vi "Robot_Control.vi"() -> ()   [LabVIEW 2014]
uses:
  <vilib>/LabVIEW Targets/FPGA/cRIO/cRIO-9505/controls.llb/_nicrio_cRIO-9505_DriveDirection.ctl
  <vilib>/Platform/TimedLoop/XDataNode/timing_clust.ctl
  <vilib>/Platform/TimedLoop/XDataNode/nitl_modes.ctl
  <vilib>/Platform/TimedLoop/XDataNode/wakeup.ctl
  <vilib>/rvi/Emulation/niFpgaGetClockAttributes.vi
  <vilib>/rvi/Emulation/niFpgaSctlEmulationGetInTimedLoop.vi
  <vilib>/rvi/Emulation/niFpgaEmulationReportErrorSimple.vi
  <vilib>/rvi/eio/common/nirviEmuTemplateMethod_errors.vi
  <vilib>/rvi/Emulation/niFpgaCriticalErrorInLSC.vi
  <vilib>/rvi/Emulation/niFpgaProcessEmulError.vi
  <vilib>/eio/EIONode/EIONode.xnode
  <vilib>/eio/EIOMethodNode/EIOMethodNode.xnode
  <vilib>/Platform/TimedLoop/XDataNode/XDataNode.xnode
  <vilib>/Platform/TimedLoop/XDataNode/XDNodeRunTimeDep.lvlib
panel:
  out "Mod1 6/Current Sense":i16
  in  "Duty Cycle 6":fxp<+,32,0>=0.5
  in  "Mod1/Drive Direction 6":T1
  out "Boolean 5":bool
  out "Boolean 4":bool
  out "Boolean 3":bool
  out "Boolean 2":bool
  out "Boolean":bool
  in  "Velocity Interval (uSec)":fxp<+/-,40,24>=5000.0
  out "Homed":bool
  in  "Duty Cycle 5":fxp<+,32,0>=0.5
  in  "Duty Cycle 4":fxp<+,32,0>=0.5
  in  "Duty Cycle 3":fxp<+,32,0>=0.5
  in  "Duty Cycle 2":fxp<+,32,0>=0.5
  in  "Duty Cycle 1":fxp<+,32,0>=0.5
  in  "Stop":bool
  in  "Mod1/Drive Direction 5":T1
  in  "Mod1/Drive Direction 4":T1=enum."Counterclockwise"
  in  "Mod1/Drive Direction 3":T1=enum."Counterclockwise"
  in  "Mod1/Drive Direction 2":T1=enum."Counterclockwise"
  in  "Mod1/Drive Direction":T1
  out "Position (Degrees) 5":fxp<+/-,40,24>
  out "Velocity (Degrees/Second) 5":fxp<+/-,40,24>
  out "Position (Degrees) 4":fxp<+/-,40,24>
  out "Velocity (Degrees/Second) 4":fxp<+/-,40,24>
  out "Position (Degrees) 3":fxp<+/-,40,24>
  out "Velocity (Degrees/Second) 3":fxp<+/-,40,24>
  out "Position (Degrees) 2":fxp<+/-,40,24>
  out "Velocity (Degrees/Second) 2":fxp<+/-,40,24>
  in  "Go":bool
  out "Velocity (Degrees/Second)":fxp<+/-,40,24>
  out "Position (Degrees)":fxp<+/-,40,24>
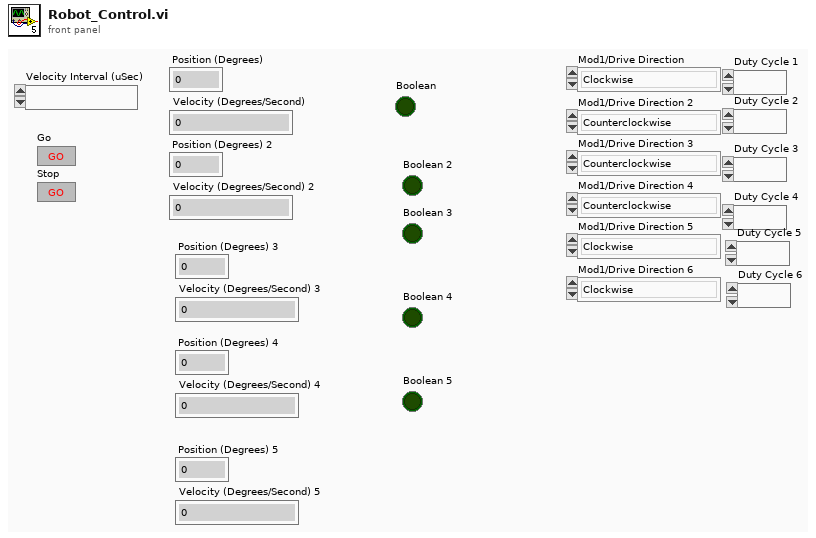
[diagram p1: front panel]
types:
  T1 = typedef "_nicrio_cRIO-9505_DriveDirection.ctl" = enum8{"Clockwise", "Counterclockwise"}
  T2 = typedef "XDNodeRunTimeDep.lvlib/timing_clust.ctl" = cluster{"Expected End [f-1]":u64, "Actual End [f-1]":u64, "Finished Late? [f-1]":bool, "Expected End [i-1]":u64, "Actual End [i-1]":u64, "Finished Late? [i-1]":bool, "Expected Start [i]":u64, "Actual Start [i]":u64, "Expected Start [f]":u64, "Actual Start [f]":u64, "Source Name":string, "Structure Name":string, "Period":i64, "Deadline":i64, "Offset":i64, "Start":i64, "Priority":i32, "Timeout":i32, "Mode":T3, "Wakeup Reason":T4, "Error":errorcluster, "Source Type":string, "Secondary Source Type":string, "Global End Time":u64, "Global Start Time":u64, "Frame Duration":u64, "Iteration Duration":u64, "Assigned CPU":i32, "I/O Scan Engine Mode":u32}
  T3 = typedef "XDNodeRunTimeDep.lvlib/nitl_modes.ctl" = enum32{"No Change", "Process missed periods, maintain original phase", "Discard missed periods, maintain original phase", "Process missed periods, ignore original phase", "Discard missed periods, ignore original phase"}
  T4 = typedef "XDNodeRunTimeDep.lvlib/wakeup.ctl" = enum32{"Normal", "Aborted", "Asynchronous wakeup", "Timing source error", "Timed loop error", "Timeout"}
  T5 = cluster{"A'":bool, "B'":bool, "Time Interval Reached":bool, "Reference Time Count":fxp<+/-,40,24>, "Previous Tick Count":fxp<+/-,40,24>, "Previous Interval Tick Count":fxp<+/-,40,24>, "Velocity":fxp<+/-,40,24>}
  T6 = cluster{"A'":bool, "B'":bool, "Time Interval Reached":bool, "Reference Time Count":fxp<+/-,64,64>, "Previous Tick Count":fxp<+/-,40,24>, "Previous Interval Tick Count":fxp<+/-,40,24>, "Velocity":fxp<+/-,40,24>}
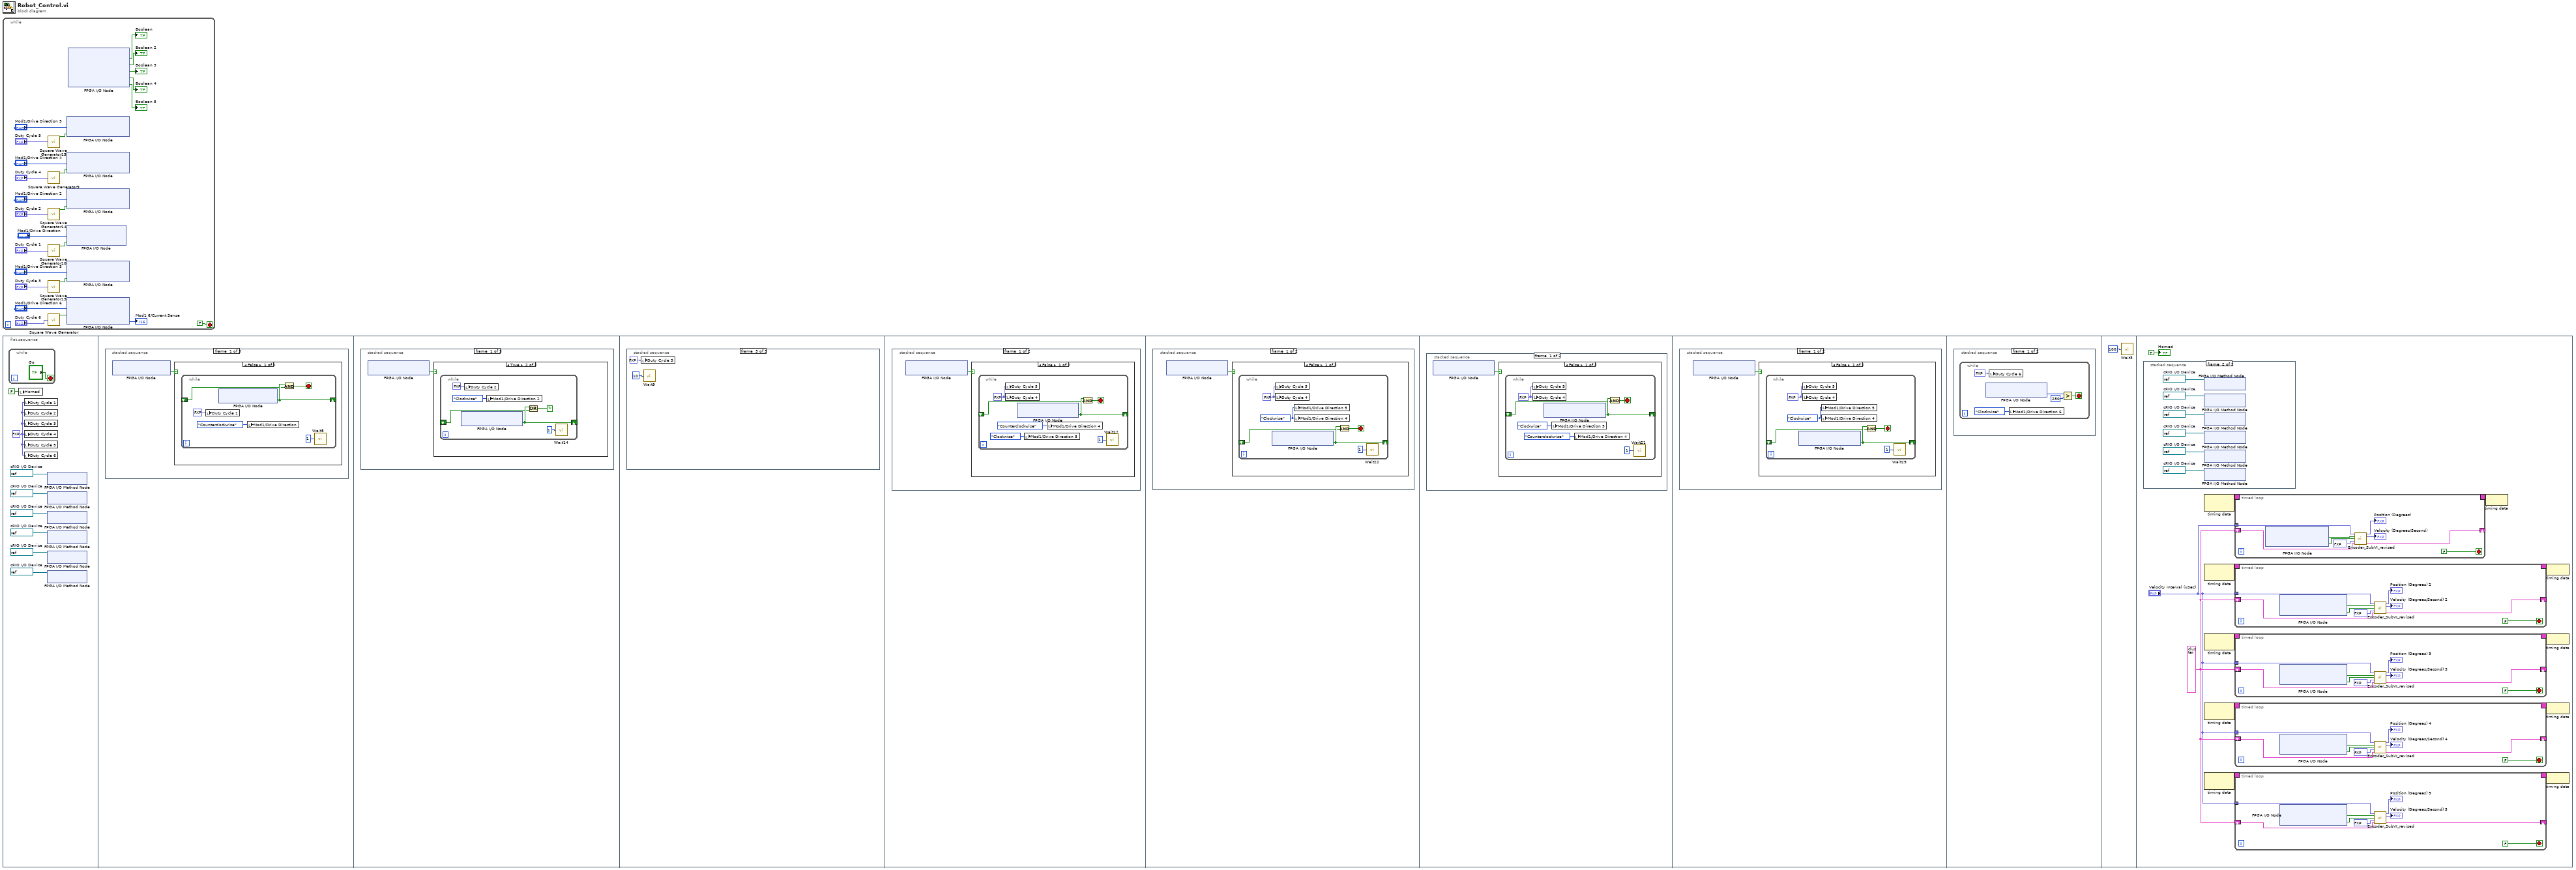
[diagram p0: block diagram]
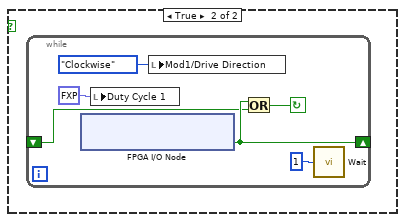
[diagram p2: hidden frame]
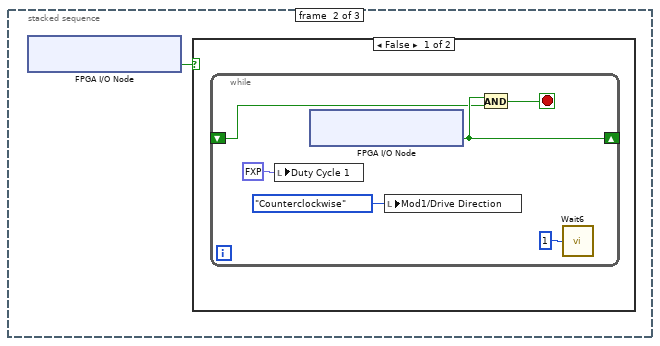
[diagram p3: hidden frame]
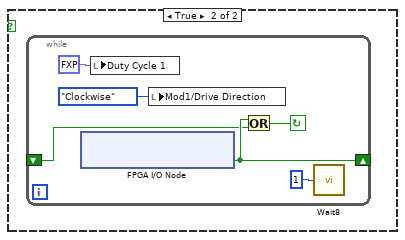
[diagram p4: hidden frame]
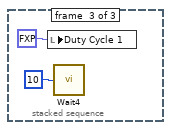
[diagram p5: hidden frame]
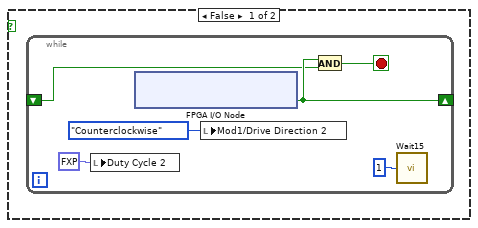
[diagram p6: hidden frame]
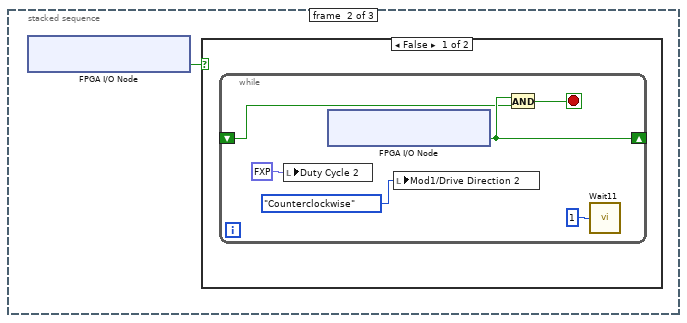
[diagram p7: hidden frame]
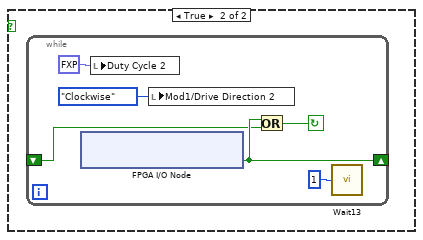
[diagram p8: hidden frame]
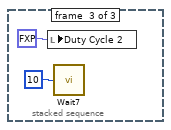
[diagram p9: hidden frame]
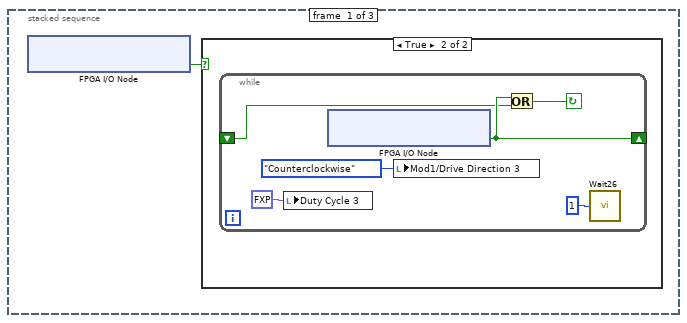
[diagram p10: hidden frame]
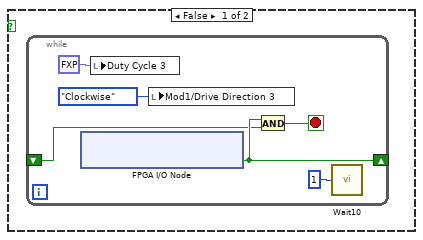
[diagram p11: hidden frame]
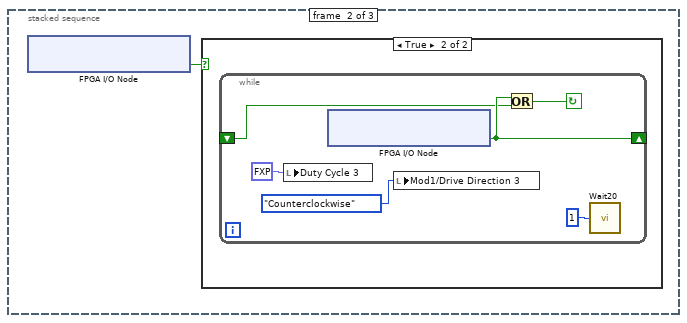
[diagram p12: hidden frame]
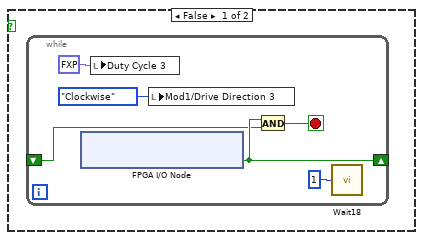
[diagram p13: hidden frame]
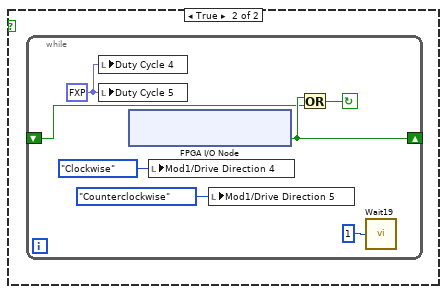
[diagram p14: hidden frame]
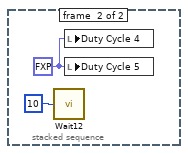
[diagram p15: hidden frame]
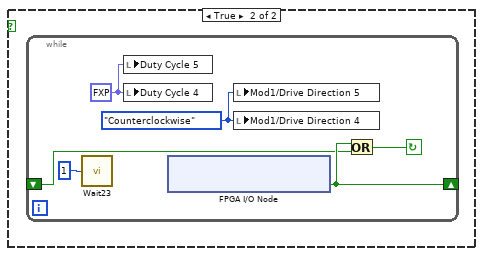
[diagram p16: hidden frame]
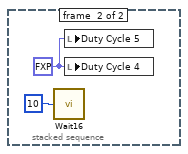
[diagram p17: hidden frame]
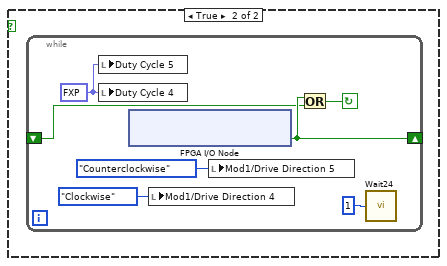
[diagram p18: hidden frame]
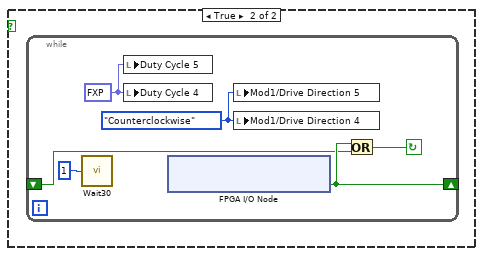
[diagram p20: hidden frame]
diagram:
  n1 = while {
    stop <- FALSE stop-if-true
    n2 = call "Square Wave Generator15"("duty cycle (periods)"="Duty Cycle 5") -> ("square wave out"=w2:bool)  [unwired: 14 in]
    n3 = call "Square Wave Generator9"("duty cycle (periods)"="Duty Cycle 4") -> ("square wave out"=w17:bool)  [unwired: 14 in]
    n4 = call "Square Wave Generator14"("duty cycle (periods)"="Duty Cycle 2") -> ("square wave out"=w3:bool)  [unwired: 14 in]
    n5 = call "Square Wave Generator10"("duty cycle (periods)"="Duty Cycle 1") -> ("square wave out"=w16:bool)  [unwired: 14 in]
    n6 = call "Square Wave Generator13"("duty cycle (periods)"="Duty Cycle 3") -> ("square wave out"=w4:bool)  [unwired: 14 in]
    n7 = call "Square Wave Generator"("duty cycle (periods)"="Duty Cycle 6") -> ("square wave out"=w18:bool)  [unwired: 14 in]
    n8 = xnode "FPGA I/O Node"("Mod1 5/Drive Direction"="Mod1/Drive Direction 5", "Mod1 5/Motor"=w2) -> ()  [unwired: 2 in, 2 out]
    n9 = xnode "FPGA I/O Node"("Mod1 4/Drive Direction"="Mod1/Drive Direction 4", "Mod1 4/Motor"=w17) -> ()  [unwired: 2 in, 2 out]
    n10 = xnode "FPGA I/O Node"("Mod1 2/Drive Direction"="Mod1/Drive Direction 2", "Mod1 2/Motor"=w3) -> ()  [unwired: 2 in, 2 out]
    n11 = xnode "FPGA I/O Node"("Mod1/Drive Direction"="Mod1/Drive Direction", "Mod1/Motor"=w16) -> ()  [unwired: 2 in, 2 out]
    n12 = xnode "FPGA I/O Node"("Mod1 3/Drive Direction"="Mod1/Drive Direction 3", "Mod1 3/Motor"=w4) -> ()  [unwired: 2 in, 2 out]
    n13 = xnode "FPGA I/O Node"("Mod1 6/Drive Direction"="Mod1/Drive Direction 6", "Mod1 6/Motor"=w18) -> ("Mod1 6/Current Sense"=→"Mod1 6/Current Sense":i16)  [unwired: 3 in, 3 out]
    n14 = xnode "FPGA I/O Node"() -> ("Mod1/Encoder Index"=→"Boolean":bool, "Mod1 2/Encoder Index"=→"Boolean 2":bool, "Mod1 3/Encoder Index"=→"Boolean 3":bool, "Mod1 4/Encoder Index"=→"Boolean 4":bool, "Mod1 5/Encoder Index"=→"Boolean 5":bool)  [unwired: 5 in, 5 out]
  }
  n15 = flat-sequence {
    frame #0 {
      w27 = refnum<k21> "Mod6"  # cRIO I/O Device
      w26 = fxp<+,32,0> 0.0 ("Duty Cycle 1")
      w31 = refnum<k21> "Mod5"  # cRIO I/O Device
      w30 = refnum<k21> "Mod4"  # cRIO I/O Device
      w29 = refnum<k21> "Mod3"  # cRIO I/O Device
      w32 = refnum<k21> "Mod2"  # cRIO I/O Device
      w33 = refnum<k21> "Mod1"  # cRIO I/O Device
      n16 = while {
        stop <- "Go" stop-if-true
      }
      n17 = local write "Homed"(FALSE ("Homed")) -> ()
      n18 = local write "Duty Cycle 1"(w26) -> ()
      n19 = local write "Duty Cycle 2"(w26) -> ()
      n20 = local write "Duty Cycle 3"(w26) -> ()
      n21 = local write "Duty Cycle 4"(w26) -> ()
      n22 = local write "Duty Cycle 5"(w26) -> ()
      n23 = local write "Duty Cycle 6"(w26) -> ()
      n24 = xnode "FPGA I/O Method Node"("FPGA I/O In"=w33) -> ()  [unwired: 1 out]
      n25 = xnode "FPGA I/O Method Node"("FPGA I/O In"=w32) -> ()  [unwired: 1 out]
      n26 = xnode "FPGA I/O Method Node"("FPGA I/O In"=w29) -> ()  [unwired: 1 out]
      n27 = xnode "FPGA I/O Method Node"("FPGA I/O In"=w30) -> ()  [unwired: 1 out]
      n28 = xnode "FPGA I/O Method Node"("FPGA I/O In"=w27) -> ()  [unwired: 1 out]
      n29 = xnode "FPGA I/O Method Node"("FPGA I/O In"=w31) -> ()  [unwired: 1 out]
    }
    frame #1 {
      n30 = stacked-sequence {
        frame #0 {
          n31 = xnode "FPGA I/O Node"() -> ("Mod1/Encoder Index"=w35:bool)  [unwired: 1 in, 1 out]
          n32 = case shown="False" w35 {
            frame False {
              n33 = while {
                shift-right: [w37] -> _
                shift-left: _ -> [w36]
                stop <- w38 stop-if-true
                n34 = local write "Duty Cycle 1"(fxp<+,32,0> 0.6999999999534339 ("phase offset (periods)")) -> ()
                n35 = xnode "FPGA I/O Node"() -> ("Mod1/Encoder Index"=w37:bool)  [unwired: 1 in, 1 out]
                n36 = local write "Mod1/Drive Direction"(_nicrio_cRIO-9505_DriveDirection."Counterclockwise" ("Mod1/Drive Direction")) -> ()
                n37 = And(x=w37, y=w36) -> (x .and. y?=w38:bool)
                n38 = call "Wait5"("Count(mSec)"=u32 1) -> ()  [unwired: 1 out]
              }
            }
            frame True {
              n39 = while {
                shift-right: [w43] -> _
                shift-left: _ -> [w42]
                stop <- w44 continue-if-true
                n40 = xnode "FPGA I/O Node"() -> ("Mod1/Encoder Index"=w43:bool)  [unwired: 1 in, 1 out]
                n41 = local write "Duty Cycle 1"(fxp<+,32,0> 0.6999999999534339 ("phase offset (periods)")) -> ()
                n42 = local write "Mod1/Drive Direction"(_nicrio_cRIO-9505_DriveDirection."Clockwise" ("Mod1/Drive Direction")) -> ()
                n43 = Or(x=w43, y=w42) -> (x .or. y?=w44:bool)
                n44 = call "Wait"("Count(mSec)"=u32 1) -> ()  [unwired: 1 out]
              }
            }
          }
        }
        frame #1 {
          n45 = xnode "FPGA I/O Node"() -> ("Mod1/Encoder Index"=w48:bool)  [unwired: 1 in, 1 out]
          n46 = case shown="False" w48 {
            frame False {
              n47 = while {
                shift-right: [w50] -> _
                shift-left: _ -> [w49]
                stop <- w51 stop-if-true
                n48 = local write "Duty Cycle 1"(fxp<+,32,0> 0.19999999995343387 ("phase offset (periods)")) -> ()
                n49 = xnode "FPGA I/O Node"() -> ("Mod1/Encoder Index"=w50:bool)  [unwired: 1 in, 1 out]
                n50 = local write "Mod1/Drive Direction"(_nicrio_cRIO-9505_DriveDirection."Counterclockwise" ("Mod1/Drive Direction")) -> ()
                n51 = And(x=w50, y=w49) -> (x .and. y?=w51:bool)
                n52 = call "Wait6"("Count(mSec)"=u32 1) -> ()  [unwired: 1 out]
              }
            }
            frame True {
              n53 = while {
                shift-right: [w56] -> _
                shift-left: _ -> [w55]
                stop <- w57 continue-if-true
                n54 = xnode "FPGA I/O Node"() -> ("Mod1/Encoder Index"=w56:bool)  [unwired: 1 in, 1 out]
                n55 = local write "Duty Cycle 1"(fxp<+,32,0> 0.19999999995343387 ("phase offset (periods)")) -> ()
                n56 = local write "Mod1/Drive Direction"(_nicrio_cRIO-9505_DriveDirection."Clockwise" ("Mod1/Drive Direction")) -> ()
                n57 = Or(x=w56, y=w55) -> (x .or. y?=w57:bool)
                n58 = call "Wait8"("Count(mSec)"=u32 1) -> ()  [unwired: 1 out]
              }
            }
          }
        }
        frame #2 {
          n59 = local write "Duty Cycle 1"(fxp<+,32,0> 0.0 ("Duty Cycle 1")) -> ()
          n60 = call "Wait4"("Count(mSec)"=u32 10) -> ()  [unwired: 1 out]
        }
      }
    }
    frame #2 {
      n61 = stacked-sequence {
        frame #0 {
          n62 = xnode "FPGA I/O Node"() -> ("Mod1 2/Encoder Index"=w63:bool)  [unwired: 1 in, 1 out]
          n63 = case shown="True" w63 {
            frame False {
              n64 = while {
                shift-right: [w65] -> _
                shift-left: _ -> [w64]
                stop <- w66 stop-if-true
                n65 = local write "Duty Cycle 2"(fxp<+,32,0> 0.6999999999534339 ("phase offset (periods)")) -> ()
                n66 = xnode "FPGA I/O Node"() -> ("Mod1 2/Encoder Index"=w65:bool)  [unwired: 1 in, 1 out]
                n67 = local write "Mod1/Drive Direction 2"(_nicrio_cRIO-9505_DriveDirection."Counterclockwise" ("Mod1/Drive Direction")) -> ()
                n68 = And(x=w65, y=w64) -> (x .and. y?=w66:bool)
                n69 = call "Wait15"("Count(mSec)"=u32 1) -> ()  [unwired: 1 out]
              }
            }
            frame True {
              n70 = while {
                shift-right: [w71] -> _
                shift-left: _ -> [w70]
                stop <- w72 continue-if-true
                n71 = xnode "FPGA I/O Node"() -> ("Mod1 2/Encoder Index"=w71:bool)  [unwired: 1 in, 1 out]
                n72 = local write "Duty Cycle 2"(fxp<+,32,0> 0.6999999999534339 ("phase offset (periods)")) -> ()
                n73 = local write "Mod1/Drive Direction 2"(_nicrio_cRIO-9505_DriveDirection."Clockwise" ("Mod1/Drive Direction")) -> ()
                n74 = Or(x=w71, y=w70) -> (x .or. y?=w72:bool)
                n75 = call "Wait14"("Count(mSec)"=u32 1) -> ()  [unwired: 1 out]
              }
            }
          }
        }
        frame #1 {
          n76 = xnode "FPGA I/O Node"() -> ("Mod1 2/Encoder Index"=w76:bool)  [unwired: 1 in, 1 out]
          n77 = case shown="False" w76 {
            frame False {
              n78 = while {
                shift-right: [w78] -> _
                shift-left: _ -> [w77]
                stop <- w79 stop-if-true
                n79 = local write "Duty Cycle 2"(fxp<+,32,0> 0.19999999995343387 ("phase offset (periods)")) -> ()
                n80 = xnode "FPGA I/O Node"() -> ("Mod1 2/Encoder Index"=w78:bool)  [unwired: 1 in, 1 out]
                n81 = local write "Mod1/Drive Direction 2"(_nicrio_cRIO-9505_DriveDirection."Counterclockwise" ("Mod1/Drive Direction")) -> ()
                n82 = And(x=w78, y=w77) -> (x .and. y?=w79:bool)
                n83 = call "Wait11"("Count(mSec)"=u32 1) -> ()  [unwired: 1 out]
              }
            }
            frame True {
              n84 = while {
                shift-right: [w84] -> _
                shift-left: _ -> [w83]
                stop <- w85 continue-if-true
                n85 = xnode "FPGA I/O Node"() -> ("Mod1 2/Encoder Index"=w84:bool)  [unwired: 1 in, 1 out]
                n86 = local write "Duty Cycle 2"(fxp<+,32,0> 0.19999999995343387 ("phase offset (periods)")) -> ()
                n87 = local write "Mod1/Drive Direction 2"(_nicrio_cRIO-9505_DriveDirection."Clockwise" ("Mod1/Drive Direction")) -> ()
                n88 = Or(x=w84, y=w83) -> (x .or. y?=w85:bool)
                n89 = call "Wait13"("Count(mSec)"=u32 1) -> ()  [unwired: 1 out]
              }
            }
          }
        }
        frame #2 {
          n90 = local write "Duty Cycle 2"(fxp<+,32,0> 0.0 ("Duty Cycle 2")) -> ()
          n91 = call "Wait7"("Count(mSec)"=u32 10) -> ()  [unwired: 1 out]
        }
      }
    }
    frame #3 {
      n92 = stacked-sequence {
        frame #0 {
          n93 = xnode "FPGA I/O Node"() -> ("Mod1 3/Encoder Index"=w91:bool)  [unwired: 1 in, 1 out]
          n94 = case shown="True" w91 {
            frame False {
              n95 = while {
                shift-right: [w93] -> _
                shift-left: _ -> [w92]
                stop <- w94 stop-if-true
                n96 = xnode "FPGA I/O Node"() -> ("Mod1 3/Encoder Index"=w93:bool)  [unwired: 1 in, 1 out]
                n97 = local write "Duty Cycle 3"(fxp<+,32,0> 0.6999999999534339 ("phase offset (periods)")) -> ()
                n98 = local write "Mod1/Drive Direction 3"(_nicrio_cRIO-9505_DriveDirection."Clockwise" ("Mod1/Drive Direction")) -> ()
                n99 = And(x=w93, y=w92) -> (x .and. y?=w94:bool)
                n100 = call "Wait10"("Count(mSec)"=u32 1) -> ()  [unwired: 1 out]
              }
            }
            frame True {
              n101 = while {
                shift-right: [w99] -> _
                shift-left: _ -> [w98]
                stop <- w100 continue-if-true
                n102 = local write "Duty Cycle 3"(fxp<+,32,0> 0.6999999999534339 ("phase offset (periods)")) -> ()
                n103 = xnode "FPGA I/O Node"() -> ("Mod1 3/Encoder Index"=w99:bool)  [unwired: 1 in, 1 out]
                n104 = local write "Mod1/Drive Direction 3"(_nicrio_cRIO-9505_DriveDirection."Counterclockwise" ("Mod1/Drive Direction")) -> ()
                n105 = Or(x=w99, y=w98) -> (x .or. y?=w100:bool)
                n106 = call "Wait26"("Count(mSec)"=u32 1) -> ()  [unwired: 1 out]
              }
            }
          }
        }
        frame #1 {
          n107 = xnode "FPGA I/O Node"() -> ("Mod1 3/Encoder Index"=w104:bool)  [unwired: 1 in, 1 out]
          n108 = case shown="True" w104 {
            frame False {
              n109 = while {
                shift-right: [w106] -> _
                shift-left: _ -> [w105]
                stop <- w107 stop-if-true
                n110 = xnode "FPGA I/O Node"() -> ("Mod1 3/Encoder Index"=w106:bool)  [unwired: 1 in, 1 out]
                n111 = local write "Duty Cycle 3"(fxp<+,32,0> 0.19999999995343387 ("phase offset (periods)")) -> ()
                n112 = local write "Mod1/Drive Direction 3"(_nicrio_cRIO-9505_DriveDirection."Clockwise" ("Mod1/Drive Direction")) -> ()
                n113 = And(x=w106, y=w105) -> (x .and. y?=w107:bool)
                n114 = call "Wait18"("Count(mSec)"=u32 1) -> ()  [unwired: 1 out]
              }
            }
            frame True {
              n115 = while {
                shift-right: [w112] -> _
                shift-left: _ -> [w111]
                stop <- w113 continue-if-true
                n116 = local write "Duty Cycle 3"(fxp<+,32,0> 0.19999999995343387 ("phase offset (periods)")) -> ()
                n117 = xnode "FPGA I/O Node"() -> ("Mod1 3/Encoder Index"=w112:bool)  [unwired: 1 in, 1 out]
                n118 = local write "Mod1/Drive Direction 3"(_nicrio_cRIO-9505_DriveDirection."Counterclockwise" ("Mod1/Drive Direction")) -> ()
                n119 = Or(x=w112, y=w111) -> (x .or. y?=w113:bool)
                n120 = call "Wait20"("Count(mSec)"=u32 1) -> ()  [unwired: 1 out]
              }
            }
          }
        }
        frame #2 {
          n121 = local write "Duty Cycle 3"(fxp<+,32,0> 0.0 ("Duty Cycle 3")) -> ()
          n122 = call "Wait9"("Count(mSec)"=u32 10) -> ()  [unwired: 1 out]
        }
      }
    }
    frame #4 {
      n123 = stacked-sequence {
        frame #0 {
          n124 = xnode "FPGA I/O Node"() -> ("Mod1 4/Encoder Index"=w119:bool)  [unwired: 1 in, 1 out]
          n125 = case shown="False" w119 {
            frame False {
              n126 = while {
                shift-right: [w121] -> _
                shift-left: _ -> [w120]
                stop <- w122 stop-if-true
                w125 = fxp<+,32,0> 0.6999999999534339 ("phase offset (periods)")
                n127 = local write "Duty Cycle 5"(w125) -> ()
                n128 = local write "Duty Cycle 4"(w125) -> ()
                n129 = xnode "FPGA I/O Node"() -> ("Mod1 4/Encoder Index"=w121:bool)  [unwired: 1 in, 1 out]
                n130 = local write "Mod1/Drive Direction 5"(_nicrio_cRIO-9505_DriveDirection."Clockwise" ("Mod1/Drive Direction")) -> ()
                n131 = local write "Mod1/Drive Direction 4"(_nicrio_cRIO-9505_DriveDirection."Counterclockwise" ("Mod1/Drive Direction")) -> ()
                n132 = And(x=w121, y=w120) -> (x .and. y?=w122:bool)
                n133 = call "Wait17"("Count(mSec)"=u32 1) -> ()  [unwired: 1 out]
              }
            }
            frame True {
              n134 = while {
                shift-right: [w128] -> _
                shift-left: _ -> [w127]
                stop <- w129 continue-if-true
                w130 = fxp<+,32,0> 0.6999999999534339 ("phase offset (periods)")
                n135 = local write "Duty Cycle 4"(w130) -> ()
                n136 = local write "Duty Cycle 5"(w130) -> ()
                n137 = xnode "FPGA I/O Node"() -> ("Mod1 4/Encoder Index"=w128:bool)  [unwired: 1 in, 1 out]
                n138 = local write "Mod1/Drive Direction 4"(_nicrio_cRIO-9505_DriveDirection."Clockwise" ("Mod1/Drive Direction")) -> ()
                n139 = local write "Mod1/Drive Direction 5"(_nicrio_cRIO-9505_DriveDirection."Counterclockwise" ("Mod1/Drive Direction")) -> ()
                n140 = Or(x=w128, y=w127) -> (x .or. y?=w129:bool)
                n141 = call "Wait19"("Count(mSec)"=u32 1) -> ()  [unwired: 1 out]
              }
            }
          }
        }
        frame #1 {
          w135 = fxp<+,32,0> 0.0 ("Duty Cycle 4")
          n142 = call "Wait12"("Count(mSec)"=u32 10) -> ()  [unwired: 1 out]
          n143 = local write "Duty Cycle 4"(w135) -> ()
          n144 = local write "Duty Cycle 5"(w135) -> ()
        }
      }
    }
    frame #5 {
      n145 = stacked-sequence {
        frame #0 {
          n146 = xnode "FPGA I/O Node"() -> ("Mod1 5/Encoder Index"=w136:bool)  [unwired: 1 in, 1 out]
          n147 = case shown="False" w136 {
            frame False {
              n148 = while {
                shift-right: [w139] -> _
                shift-left: _ -> [w137]
                stop <- w138 stop-if-true
                w140 = fxp<+,32,0> 0.6999999999534339 ("phase offset (periods)")
                w142 = _nicrio_cRIO-9505_DriveDirection."Clockwise" ("Mod1/Drive Direction")
                n149 = xnode "FPGA I/O Node"() -> ("Mod1 5/Encoder Index"=w139:bool)  [unwired: 1 in, 1 out]
                n150 = local write "Duty Cycle 5"(w140) -> ()
                n151 = local write "Duty Cycle 4"(w140) -> ()
                n152 = local write "Mod1/Drive Direction 5"(w142) -> ()
                n153 = local write "Mod1/Drive Direction 4"(w142) -> ()
                n154 = And(x=w139, y=w137) -> (x .and. y?=w138:bool)
                n155 = call "Wait22"("Count(mSec)"=u32 1) -> ()  [unwired: 1 out]
              }
            }
            frame True {
              n156 = while {
                shift-right: [w144] -> _
                shift-left: _ -> [w143]
                stop <- w145 continue-if-true
                w146 = fxp<+,32,0> 0.6999999999534339 ("phase offset (periods)")
                w148 = _nicrio_cRIO-9505_DriveDirection."Counterclockwise" ("Mod1/Drive Direction")
                n157 = call "Wait23"("Count(mSec)"=u32 1) -> ()  [unwired: 1 out]
                n158 = local write "Duty Cycle 5"(w146) -> ()
                n159 = local write "Duty Cycle 4"(w146) -> ()
                n160 = xnode "FPGA I/O Node"() -> ("Mod1 5/Encoder Index"=w144:bool)  [unwired: 1 in, 1 out]
                n161 = local write "Mod1/Drive Direction 5"(w148) -> ()
                n162 = local write "Mod1/Drive Direction 4"(w148) -> ()
                n163 = Or(x=w144, y=w143) -> (x .or. y?=w145:bool)
              }
            }
          }
        }
        frame #1 {
          w150 = fxp<+,32,0> 0.0 ("Duty Cycle 4")
          n164 = call "Wait16"("Count(mSec)"=u32 10) -> ()  [unwired: 1 out]
          n165 = local write "Duty Cycle 5"(w150) -> ()
          n166 = local write "Duty Cycle 4"(w150) -> ()
        }
      }
    }
    frame #6 {
      n167 = stacked-sequence {
        frame #0 {
          n168 = xnode "FPGA I/O Node"() -> ("Mod1 4/Encoder Index"=w151:bool)  [unwired: 1 in, 1 out]
          n169 = case shown="False" w151 {
            frame False {
              n170 = while {
                shift-right: [w153] -> _
                shift-left: _ -> [w152]
                stop <- w154 stop-if-true
                w157 = fxp<+,32,0> 0.25 ("phase offset (periods)")
                n171 = local write "Duty Cycle 5"(w157) -> ()
                n172 = local write "Duty Cycle 4"(w157) -> ()
                n173 = xnode "FPGA I/O Node"() -> ("Mod1 4/Encoder Index"=w153:bool)  [unwired: 1 in, 1 out]
                n174 = local write "Mod1/Drive Direction 5"(_nicrio_cRIO-9505_DriveDirection."Clockwise" ("Mod1/Drive Direction")) -> ()
                n175 = local write "Mod1/Drive Direction 4"(_nicrio_cRIO-9505_DriveDirection."Counterclockwise" ("Mod1/Drive Direction")) -> ()
                n176 = And(x=w153, y=w152) -> (x .and. y?=w154:bool)
                n177 = call "Wait21"("Count(mSec)"=u32 1) -> ()  [unwired: 1 out]
              }
            }
            frame True {
              n178 = while {
                shift-right: [w160] -> _
                shift-left: _ -> [w159]
                stop <- w161 continue-if-true
                w164 = fxp<+,32,0> 0.25 ("phase offset (periods)")
                n179 = local write "Duty Cycle 5"(w164) -> ()
                n180 = local write "Duty Cycle 4"(w164) -> ()
                n181 = xnode "FPGA I/O Node"() -> ("Mod1 4/Encoder Index"=w160:bool)  [unwired: 1 in, 1 out]
                n182 = local write "Mod1/Drive Direction 4"(_nicrio_cRIO-9505_DriveDirection."Clockwise" ("Mod1/Drive Direction")) -> ()
                n183 = local write "Mod1/Drive Direction 5"(_nicrio_cRIO-9505_DriveDirection."Counterclockwise" ("Mod1/Drive Direction")) -> ()
                n184 = Or(x=w160, y=w159) -> (x .or. y?=w161:bool)
                n185 = call "Wait24"("Count(mSec)"=u32 1) -> ()  [unwired: 1 out]
              }
            }
          }
        }
        frame #1 {
        }
      }
    }
    frame #7 {
      n186 = stacked-sequence {
        frame #0 {
          n187 = xnode "FPGA I/O Node"() -> ("Mod1 5/Encoder Index"=w166:bool)  [unwired: 1 in, 1 out]
          n188 = case shown="False" w166 {
            frame False {
              n189 = while {
                shift-right: [w168] -> _
                shift-left: _ -> [w167]
                stop <- w169 stop-if-true
                w171 = fxp<+,32,0> 0.25 ("duty cycle (periods)")
                w172 = _nicrio_cRIO-9505_DriveDirection."Clockwise" ("Mod1/Drive Direction")
                n190 = xnode "FPGA I/O Node"() -> ("Mod1 5/Encoder Index"=w168:bool)  [unwired: 1 in, 1 out]
                n191 = local write "Duty Cycle 5"(w171) -> ()
                n192 = local write "Duty Cycle 4"(w171) -> ()
                n193 = local write "Mod1/Drive Direction 5"(w172) -> ()
                n194 = local write "Mod1/Drive Direction 4"(w172) -> ()
                n195 = And(x=w168, y=w167) -> (x .and. y?=w169:bool)
                n196 = call "Wait29"("Count(mSec)"=u32 1) -> ()  [unwired: 1 out]
              }
            }
            frame True {
              n197 = while {
                shift-right: [w174] -> _
                shift-left: _ -> [w173]
                stop <- w175 continue-if-true
                w177 = fxp<+,32,0> 0.25 ("duty cycle (periods)")
                w178 = _nicrio_cRIO-9505_DriveDirection."Counterclockwise" ("Mod1/Drive Direction")
                n198 = call "Wait30"("Count(mSec)"=u32 1) -> ()  [unwired: 1 out]
                n199 = local write "Duty Cycle 5"(w177) -> ()
                n200 = local write "Duty Cycle 4"(w177) -> ()
                n201 = xnode "FPGA I/O Node"() -> ("Mod1 5/Encoder Index"=w174:bool)  [unwired: 1 in, 1 out]
                n202 = local write "Mod1/Drive Direction 5"(w178) -> ()
                n203 = local write "Mod1/Drive Direction 4"(w178) -> ()
                n204 = Or(x=w174, y=w173) -> (x .or. y?=w175:bool)
              }
            }
          }
        }
        frame #1 {
          w180 = fxp<+,32,0> 0.0 ("Duty Cycle 4")
          n205 = call "Wait34"("Count(mSec)"=u32 10) -> ()  [unwired: 1 out]
          n206 = local write "Duty Cycle 5"(w180) -> ()
          n207 = local write "Duty Cycle 4"(w180) -> ()
        }
      }
    }
    frame #8 {
      n208 = stacked-sequence {
        frame #0 {
          n209 = while {
            stop <- w183 stop-if-true
            n210 = xnode "FPGA I/O Node"() -> ("Mod1 6/Current Sense"=w185:i16)  [unwired: 1 in, 1 out]
            n211 = local write "Duty Cycle 6"(fxp<+,32,0> 0.25 ("duty cycle (periods)")) -> ()
            n212 = local write "Mod1/Drive Direction 6"(_nicrio_cRIO-9505_DriveDirection."Clockwise" ("Mod1/Drive Direction")) -> ()
            n213 = Greater?(x=w185, y=i16 250) -> (0:w183:bool)
          }
        }
        frame #1 {
          n214 = local write "Duty Cycle 6"(fxp<+,32,0> 0.0 ("Duty Cycle 4")) -> ()
          n215 = call "Wait25"("Count(mSec)"=u32 10) -> ()  [unwired: 1 out]
        }
      }
    }
    frame #9 {
      n216 = call "Wait3"("Count(mSec)"=u32 100) -> ()  [unwired: 1 out]
    }
    frame #10 {
      w190 = T5 {"A'"=FALSE, "B'"=FALSE, "Time Interval Reached"=FALSE, "Reference Time Count"=0.0, "Previous Tick Count"=0.0, "Previous Interval Tick Count"=0.0, "Velocity"=0.0} ("Previous Variables Input")
      n217 = stacked-sequence {
        frame #0 {
          n218 = while {
            stop <- "Stop" stop-if-true
          }
        }
        frame #1 {
          w208 = refnum<k21> "Mod6"  # cRIO I/O Device
          w204 = refnum<k21> "Mod5"  # cRIO I/O Device
          w205 = refnum<k21> "Mod4"  # cRIO I/O Device
          w203 = refnum<k21> "Mod3"  # cRIO I/O Device
          w206 = refnum<k21> "Mod2"  # cRIO I/O Device
          w207 = refnum<k21> "Mod1"  # cRIO I/O Device
          n219 = xnode "FPGA I/O Method Node"("FPGA I/O In"=w204) -> ()  [unwired: 1 out]
          n220 = xnode "FPGA I/O Method Node"("FPGA I/O In"=w208) -> ()  [unwired: 1 out]
          n221 = xnode "FPGA I/O Method Node"("FPGA I/O In"=w206) -> ()  [unwired: 1 out]
          n222 = xnode "FPGA I/O Method Node"("FPGA I/O In"=w207) -> ()  [unwired: 1 out]
          n223 = xnode "FPGA I/O Method Node"("FPGA I/O In"=w205) -> ()  [unwired: 1 out]
          n224 = xnode "FPGA I/O Method Node"("FPGA I/O In"=w203) -> ()  [unwired: 1 out]
        }
      }
      n225 = node-c288() -> (w200:T2)  [unwired: 1 in]
      n226 = node-c288() -> (w198:T2)  [unwired: 1 in]
      n227 = node-c288() -> (w196:T2)  [unwired: 1 in]
      n228 = node-c288() -> (w194:T2)  [unwired: 1 in]
      n229 = node-c288() -> (w192:T2)  [unwired: 1 in]
      n230 = timed-loop {
        timing: w200 -> [_]
        timing-out: [_] -> w199
        shift-right: [w266] -> _
        shift-left: w190 -> [w261]
        tunnel: "Velocity Interval (uSec)" -> [w265]
        stop <- FALSE stop-if-true
        n231 = xnode "FPGA I/O Node"() -> ("Mod1/Encoder Phase A"=w264:bool, "Mod1/Encoder Phase B"=w263:bool)  [unwired: 2 in, 2 out]
        n232 = call "Encoder_SubVI_revised.vi"("Velocity Interval (uSec)"=w265, "A"=w264, "B"=w263, "Encoder Ticks Per Revolution"=fxp<+/-,40,24> 51080.0, "Previous Variables Input"=w261) -> ("Position (Degrees)"=→"Position (Degrees)":fxp<+/-,40,24>, "Velocity (Degrees/Second)"=→"Velocity (Degrees/Second)":fxp<+/-,40,24>, "Previous Variables Output"=w266:T6)  [unwired: 8 in]
      }
      n233 = timed-loop {
        timing: w198 -> [_]
        timing-out: [_] -> w197
        shift-right: [w250] -> _
        shift-left: w190 -> [w251]
        tunnel: "Velocity Interval (uSec)" -> [w249]
        stop <- FALSE stop-if-true
        n234 = xnode "FPGA I/O Node"() -> ("Mod1 2/Encoder Phase A"=w254:bool, "Mod1 2/Encoder Phase B"=w253:bool)  [unwired: 2 in, 2 out]
        n235 = call "Encoder_SubVI_revised.vi"("Velocity Interval (uSec)"=w249, "A"=w254, "B"=w253, "Encoder Ticks Per Revolution"=fxp<+/-,40,24> 40864.0 ("Encoder Ticks Per Revolution 2"), "Previous Variables Input"=w251) -> ("Position (Degrees)"=→"Position (Degrees) 2":fxp<+/-,40,24>, "Velocity (Degrees/Second)"=→"Velocity (Degrees/Second) 2":fxp<+/-,40,24>, "Previous Variables Output"=w250:T6)  [unwired: 8 in]
      }
      n236 = timed-loop {
        timing: w196 -> [_]
        timing-out: [_] -> w195
        shift-right: [w237] -> _
        shift-left: w190 -> [w238]
        tunnel: "Velocity Interval (uSec)" -> [w236]
        stop <- FALSE stop-if-true
        n237 = xnode "FPGA I/O Node"() -> ("Mod1 3/Encoder Phase A"=w240:bool, "Mod1 3/Encoder Phase B"=w239:bool)  [unwired: 2 in, 2 out]
        n238 = call "Encoder_SubVI_revised.vi"("Velocity Interval (uSec)"=w236, "A"=w240, "B"=w239, "Encoder Ticks Per Revolution"=fxp<+/-,40,24> 40864.0 ("Encoder Ticks Per Revolution 2"), "Previous Variables Input"=w238) -> ("Position (Degrees)"=→"Position (Degrees) 3":fxp<+/-,40,24>, "Velocity (Degrees/Second)"=→"Velocity (Degrees/Second) 3":fxp<+/-,40,24>, "Previous Variables Output"=w237:T6)  [unwired: 8 in]
      }
      n239 = timed-loop {
        timing: w194 -> [_]
        timing-out: [_] -> w193
        shift-right: [w224] -> _
        shift-left: w190 -> [w225]
        tunnel: "Velocity Interval (uSec)" -> [w223]
        stop <- FALSE stop-if-true
        n240 = xnode "FPGA I/O Node"() -> ("Mod1 4/Encoder Phase A"=w227:bool, "Mod1 4/Encoder Phase B"=w226:bool)  [unwired: 2 in, 2 out]
        n241 = call "Encoder_SubVI_revised.vi"("Velocity Interval (uSec)"=w223, "A"=w227, "B"=w226, "Encoder Ticks Per Revolution"=fxp<+/-,40,24> 10044.0 ("Encoder Ticks Per Revolution 4"), "Previous Variables Input"=w225) -> ("Position (Degrees)"=→"Position (Degrees) 4":fxp<+/-,40,24>, "Velocity (Degrees/Second)"=→"Velocity (Degrees/Second) 4":fxp<+/-,40,24>, "Previous Variables Output"=w224:T6)  [unwired: 8 in]
      }
      n242 = timed-loop {
        timing: w192 -> [_]
        timing-out: [_] -> w191
        shift-right: [w211] -> _
        shift-left: w190 -> [w212]
        tunnel: "Velocity Interval (uSec)" -> [w210]
        stop <- FALSE stop-if-true
        n243 = xnode "FPGA I/O Node"() -> ("Mod1 5/Encoder Phase A"=w214:bool, "Mod1 5/Encoder Phase B"=w213:bool)  [unwired: 2 in, 2 out]
        n244 = call "Encoder_SubVI_revised.vi"("Velocity Interval (uSec)"=w210, "A"=w214, "B"=w213, "Encoder Ticks Per Revolution"=fxp<+/-,40,24> 10044.0 ("Encoder Ticks Per Revolution 4"), "Previous Variables Input"=w212) -> ("Position (Degrees)"=→"Position (Degrees) 5":fxp<+/-,40,24>, "Velocity (Degrees/Second)"=→"Velocity (Degrees/Second) 5":fxp<+/-,40,24>, "Previous Variables Output"=w211:T6)  [unwired: 8 in]
      }
      n245 = node-c288(w199) -> ()
      n246 = node-c288(w197) -> ()
      n247 = node-c288(w195) -> ()
      n248 = node-c288(w193) -> ()
      n249 = node-c288(w191) -> ()
      "Homed" <- TRUE ("Homed")
    }
  }
